vi "dfd_Lattice ARMA Normalization (Basic).vi"(7 "scale type":T1, 9 "coefficients v":dbl[](array[numeric]) format="%.2f", 10 "coefficients k":dbl[](array[numeric]) format="%.2f", 11 "x":dbl[](array[numeric])) -> (2 "norm":dbl[](array[numeric]) format="%.2f", 3 "y":dbl[](array[numeric]))   [LabVIEW 2017, in "NI_DigFilter_FXP.lvlib"]
uses:
  <vilib>/addons/Digital Filter Design/NI_DigFilter_FXP.lvlib
  <vilib>/addons/Digital Filter Design/_Objects.llb/DFD Coef Norm Type.ctl
  <vilib>/addons/Digital Filter Design/NI_DigFilterLicensed.lvlib
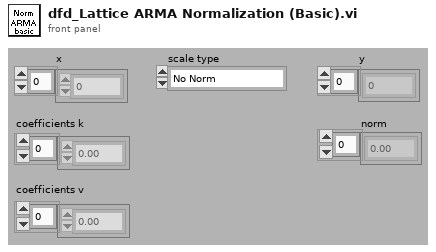
[diagram p1: front panel]
types:
  T1 = typedef "NI_DigFilterLicensed.lvlib/DFD Coef Norm Type.ctl" = enum16{"No Norm", "Time Domain 1-Norm", "Time Domain 2-Norm", "Time Domain Inf-Norm"}
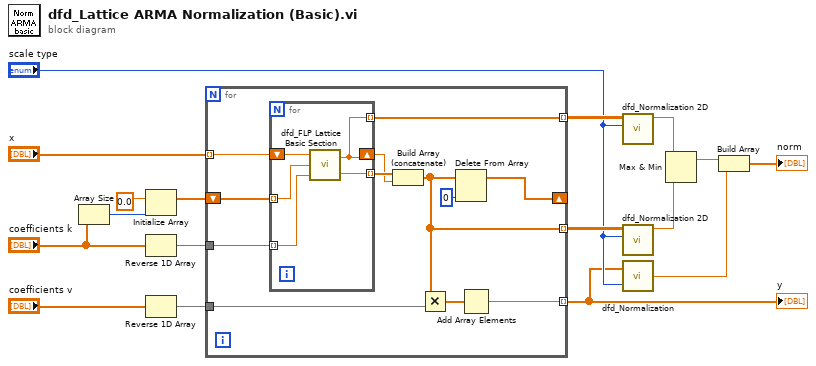
[diagram p0: block diagram]
diagram:
  n1 = Array Size(array="coefficients k") -> (size(s)=w16:i32)
  n2 = Initialize Array(0.0 ("element"), w16) -> (w17:dbl[])
  n3 = Reverse 1D Array(array="coefficients k") -> (reversed array=w15:dbl[])
  n4 = Reverse 1D Array(array="coefficients v") -> (reversed array=w14:dbl[])
  n5 = for {
    tunnel: w15 -> [w29]
    shift-right: [w24] -> _
    shift-left: w17 -> [w28]
    tunnel: [w18] -> w2 mode=indexing
    tunnel: w14 -> [w23]
    tunnel: [w22] -> w8 mode=indexing
    tunnel: [w21] -> w7 mode=indexing
    tunnel: "x" -> [w20] mode=indexing
    n6 = for {
      shift-right: [w30] -> w26
      shift-left: w20 -> [w34]
      tunnel: w28 -> [w33] mode=indexing
      tunnel: w29 -> [w32] mode=indexing
      tunnel: [w31] -> w27 mode=indexing
      tunnel: [w30] -> w22 mode=indexing
      n7 = call <vilib>:"dfd_FLP Lattice Basic Section.vi"("k(m)"=w32, "w(m-1)"=w33, "x(m)"=w34) -> ("w(m)"=w31:dbl, "x(m-1)"=w30:dbl)
    }
    n8 = Build Array (concatenate)(w27, w26) -> (w21:dbl[])
    n9 = Multiply(x=w21, y=w23) -> (x*y=w19:dbl[])
    n10 = Delete From Array(array=w21, index=0) -> (array with subset deleted=w24:dbl[])  [unwired: 1 in, 1 out]
    n11 = Add Array Elements(numeric array=w19) -> (sum=w18:dbl)
  }
  "y" <- w2
  n12 = call <vilib>:"dfd_Normalization 2D.vi"("scale type"="scale type", "2D Array (col-major)"=w8) -> ("max norm"=w6:dbl)  [unwired: 9 out]
  n13 = call <vilib>:"dfd_Normalization 2D.vi"("scale type"="scale type", "2D Array (col-major)"=w7) -> ("max norm"=w5:dbl)  [unwired: 9 out]
  n14 = call <vilib>:"dfd_Normalization.vi"("scale type"="scale type", "h(n)"=w2) -> ("norm"=w11:dbl)
  n15 = Max & Min(x=w6, y=w5) -> (max(x,y)=w3:dbl)  [unwired: 1 out]
  n16 = Build Array(w3, w11) -> (→"norm":dbl[])
